vi "RxChannel - Create Rx Channel Configuration.vi"(8 "error in (no error)":errorcluster, 11 "Parent Packet Ref":T1 format="%.0x") -> (0 "error out":errorcluster, 2 "Channel Config Ref":T1 format="%.0x")   [LabVIEW 2016, in "UDP-Custom-Device System Explorer.lvlib"]
uses:
  UDP-Custom-Device System Explorer.lvlib
  <vilib>/NI Veristand/Custom Device API/Custom Device Item Ref.ctl
  Shared/Constants.vi
  <vilib>/NI VeriStand/Custom Device API/Custom Device API.lvlib
  Shared/UDP-Custom-Device Shared.lvlib
  Property Accessors/Shared Channel Accessors.lvlib
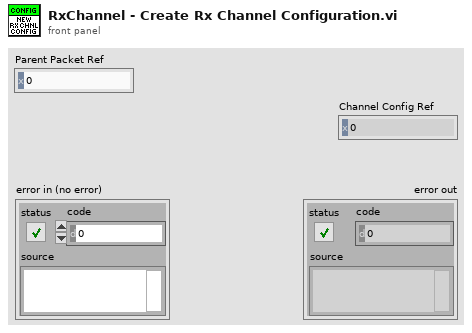
[diagram p1: front panel]
types:
  T1 = typedef "Custom Device API.lvlib/Custom Device Item Ref.ctl" = u64
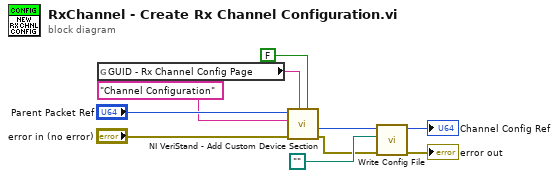
[diagram p0: block diagram]
diagram:
  n1 = global read "Constants.vi" "GUID - Rx Channel Config Page"() -> (w7:string)
  n2 = call <vilib>:"NI VeriStand - Add Custom Device Section.vi"("Highlight? (F)"=FALSE, "GUID (Default Section)"=w7, "error in (no error)"="error in (no error)", "Section Name"="Channel Configuration", "Parent Ref in"="Parent Packet Ref") -> ("error out"=w3:errorcluster, "Section Ptr"=w5:T1)  [unwired: 3 in, 2 out]
  n3 = call "Write Config File.vi"("error in (no error)"=w3, "Config File"=path "", "Node Ptr"=w5) -> ("error out"=→"error out":errorcluster, "Node Ptr out"=→"Channel Config Ref":T1)  [unwired: 7 in]
